vi "SendJSON.vi"(10 "IP Address":string, 11 "JSON in":string) -> (2 "Response Out":string, 3 "Command Out":string)   [LabVIEW 2013]
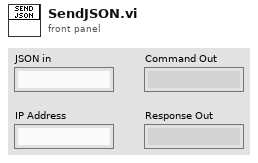
[diagram p1: front panel]
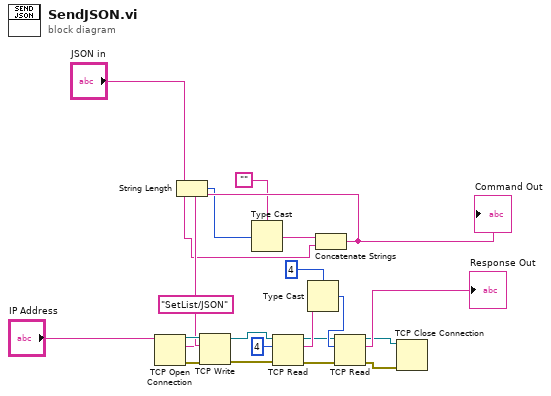
[diagram p0: block diagram]
diagram:
  n1 = TCP Open Connection(address="IP Address", remote port or service name="SetList/JSON") -> (connection ID=w8:refnum<k5>, error out=w9:errorcluster)  [unwired: 3 in]
  n2 = String Length(string="JSON in") -> (length=w3:i32)
  n3 = Type Cast(type="", x=w3) -> (*(type *) &x=w5:string)
  n4 = Concatenate Strings(w5, "JSON in") -> (w7:string)
  "Command Out" <- w7
  n5 = TCP Write(connection ID=w8, data in=w7, error in (no error)=w9) -> (connection ID out=w12:refnum<k5>, error out=w11:errorcluster)  [unwired: 1 in, 1 out]
  n6 = TCP Read(connection ID=w12, bytes to read=4, error in (no error)=w11) -> (connection ID out=w16:refnum<k5>, data out=w17:string, error out=w13:errorcluster)  [unwired: 2 in]
  n7 = Type Cast(type=4 ("bytes to read"), x=w17) -> (*(type *) &x=w18:i32)
  n8 = TCP Read(connection ID=w16, bytes to read=w18, error in (no error)=w13) -> (connection ID out=w15:refnum<k5>, data out=→"Response Out":string, error out=w14:errorcluster)  [unwired: 2 in]
  n9 = TCP Close Connection(connection ID=w15, error in (no error)=w14) -> ()  [unwired: 1 in, 2 out]
